vi "LIN EX Get Vbat Value.vi"(10 "pBatValue":u16, 11 "DevHandle":i32) -> (2 "pBatValue out":u16, 3 "function return":i32)   [LabVIEW 2010, in "usb2lin_ex.lvlib"]
doc: "int WINAPI LIN_EX_GetVbatValue(int DevHandle,unsigned short *pBatValue);"
uses:
  usb2lin_ex.lvlib
  USB2XXX.dll
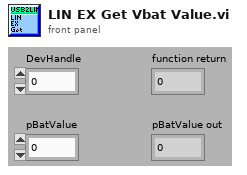
[diagram p1: front panel]
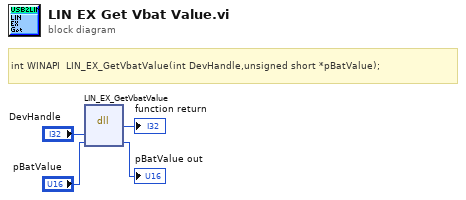
[diagram p0: block diagram]
diagram:
  # "int WINAPI  LIN_EX_GetVbatValue(int DevHandle,unsigned short *pBatValue);"
  n1 = dll-call lib="E:/OtherWork/STM32/USB2XXX_Example/trunk/SDK/api/Labview/USB2XXX.*" fn="LIN_EX_GetVbatValue"("DevHandle"="DevHandle", "pBatValue"="pBatValue") -> (→"function return":i32, "pBatValue"=→"pBatValue out":u16)  [unwired: 4 in, 2 out]
